vi "Laboratory_practice3.vi"() -> ()   [LabVIEW 2022 SP3]
panel:
  in  "Wait time":dbl
  out "Count":dbl
  in  "Number of repetitions":i16
  in  "Multiple":dbl
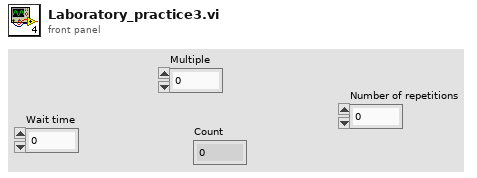
[diagram p1: front panel]
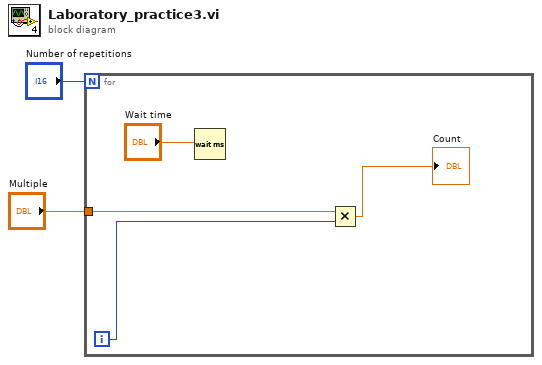
[diagram p0: block diagram]
diagram:
  n1 = for {
    N: "Number of repetitions" -> [_]
    tunnel: "Multiple" -> [w6]
    i -> [w5]
    n2 = Wait (ms)(milliseconds to wait="Wait time") -> ()  [unwired: 1 out]
    n3 = Multiply(x=w6, y=w5) -> (x*y=→"Count":dbl)
  }
